vi "test_RPLiDAR_unit-cmd-tester.vi"() -> ()   [LabVIEW 2019]
uses:
  <vilib>/Instr/_visa.llb/VISA Configure Serial Port (Instr).vi
panel:
  out "Waveform Chart":u32(graph)
  out "error out":errorcluster
  in  "clear":bool
  in  "unsigned byte array 9":u8[](array[numeric])=[165, 130, 5, 0, 0, 0, 0, 0, 34] format="%02x"
  in  "unsigned byte array 10":u8[](array[numeric])=[165, 37, 165, 240, 2, 0, 0, 87, 165, 37, 0, 0, 0, 0, 0, 0, 0, 0, 0, 0, 0, 0, 0, 0, 0, 0, 0, 0, 0, 0, 0, 0, 0, 0, 0, 0, 0, 121] format="%02x"
  in  "write 10":bool
  in  "write 9":bool
  in  "84 get lidar conf":u8[](array[numeric])=[165, 132, 36, 117, 0, 0, 0, 1, 0, 0, 0, 0, 0, 0, 0, 0, 0, 0, 0, 0, 0, 0, 0, 0, 0, 0, 0, 0, 0, 0, 0, 0, 0, 0, 0, 0, 0, 0, 113] format="%02x"
  in  "write 8":bool
  in  "25 stop / 50 info":u8[](array[numeric])=[165, 37, 165, 80] format="%02x"
  in  "write 7":bool
  in  "84 get lidar conf":u8[](array[numeric])=[165, 132, 36, 124, 0, 0, 0, 0, 0, 0, 0, 0, 0, 0, 0, 0, 0, 0, 0, 0, 0, 0, 0, 0, 0, 0, 0, 0, 0, 0, 0, 0, 0, 0, 0, 0, 0, 0, 121] format="%02x"
  in  "write 6":bool
  in  "20 get info":u8[](array[numeric])=[165, 80] format="%02x"
  in  "write 5":bool
  in  "motor start":u8[](array[numeric])=[165, 240, 2, 148, 2, 193, 165, 80] format="%02x"
  in  "write 4":bool
  in  "write 3":bool
  in  "get health":u8[](array[numeric])=[165, 82] format="%02x"
  in  "motor stop":u8[](array[numeric])=[165, 240, 2, 0, 0, 87, 165, 80] format="%02x"
  in  "write 2":bool
  in  "dt":u32=10
  in  "write":bool
  in  "unsigned byte array":u8[](array[numeric])=[165, 255, 4, 0, 0, 0, 0, 94] format="%02x"
  out "concatenated string":string
  out "read buffer":string
  in  "stop":bool
  in  "baud rate":u32=115200
  in  "port":refnum<visa-resource-name>="COM6"
  # "A5 20\nA5 52"
  # "RPLidar command tester"
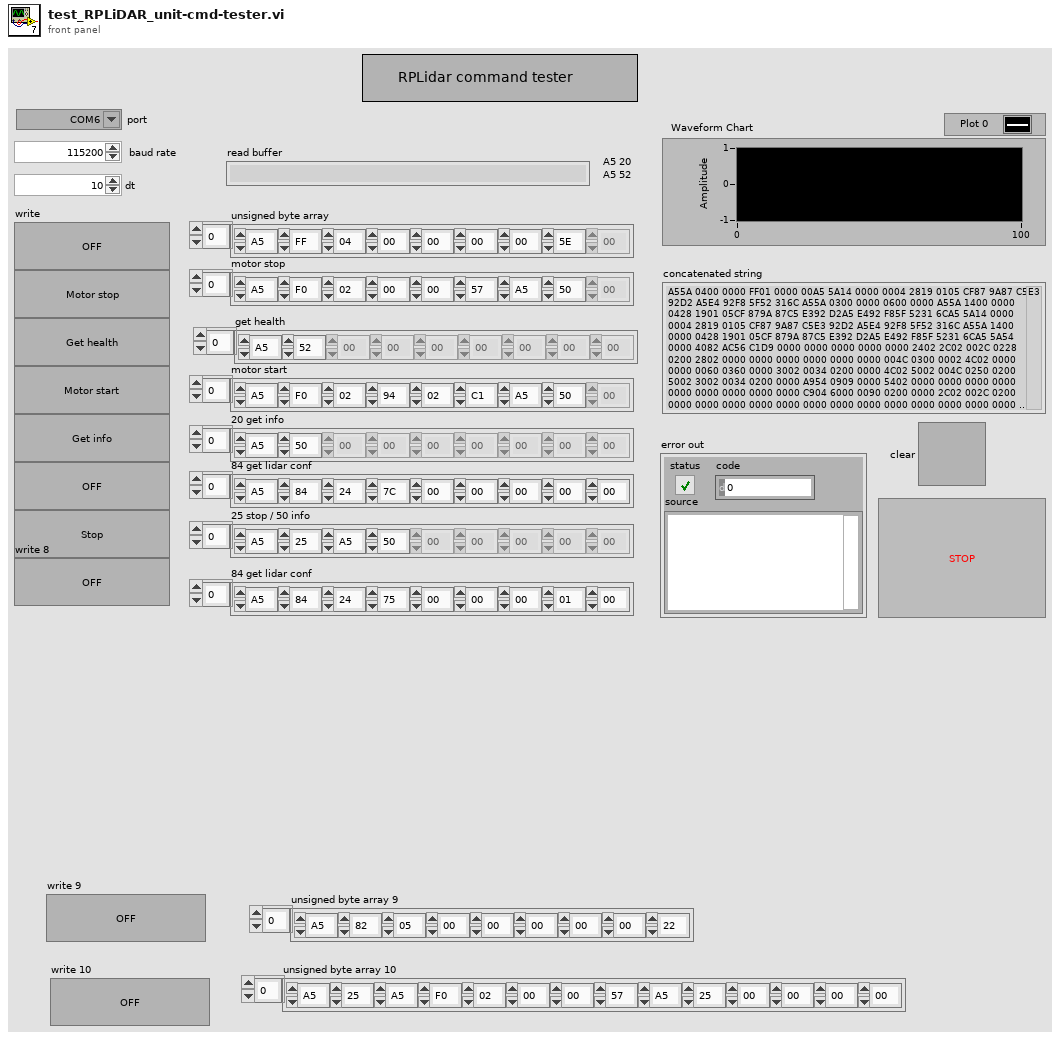
[diagram p1: front panel]
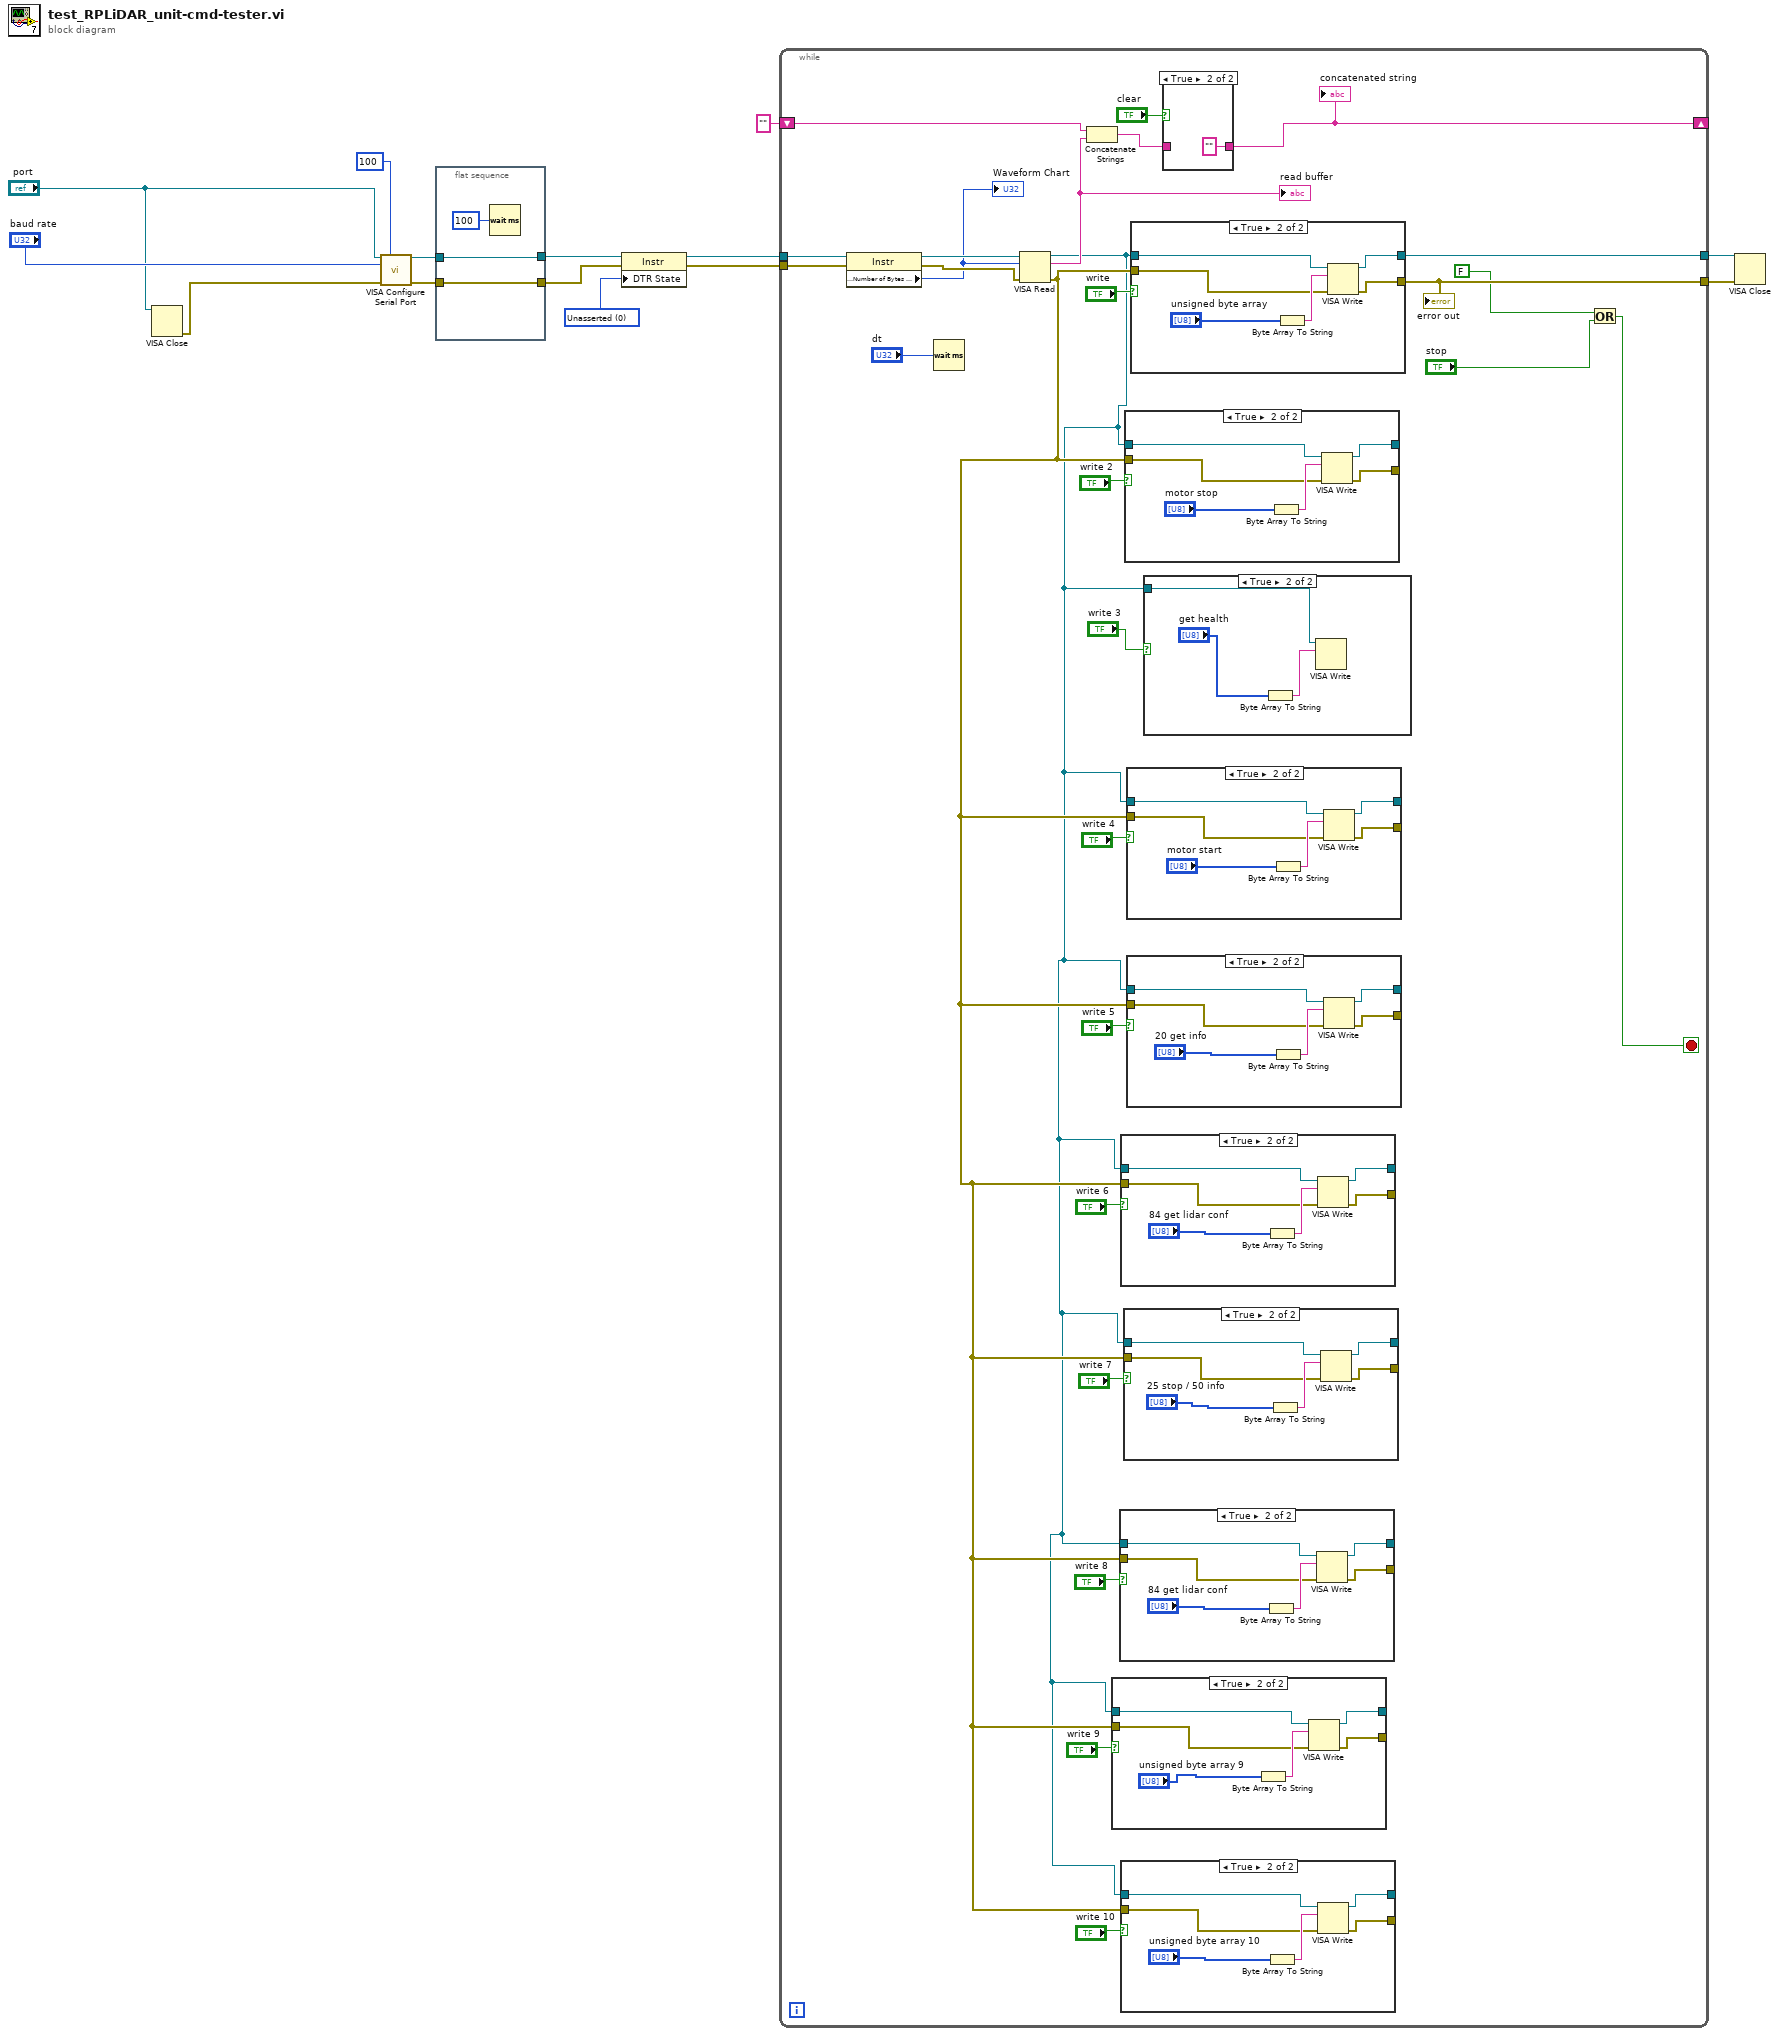
[diagram p0: block diagram]
diagram:
  w9 = i16 0 items=["Unknown"=-1, "Unasserted"=0, "Asserted"=1] ("Serial Settings:Modem Line Settings:Line DTR State")
  n1 = VISA Close(VISA resource name="port") -> (error out=w1:errorcluster)  [unwired: 1 in]
  n2 = call-poly "VISA Configure Serial Port"("VISA resource name"="port", "timeout (10sec)"=u32 100, "baud rate (9600)"="baud rate", "error in (no error)"=w1) -> ("VISA resource name out"=w13:refnum<visa-resource-name>, "error out"=w12:errorcluster)  [unwired: 10 in]
  n3 = flat-sequence {
    tunnel: [w16] -> w11
    tunnel: w13 -> [w16]
    tunnel: [w15] -> w10
    tunnel: w12 -> [w15]
    frame #0 {
      n4 = Wait (ms)(milliseconds to wait=u32 100) -> ()  [unwired: 1 out]
    }
  }
  n5 = property class="Instr"(reference=w11, error in=w10, "DTR State"=w9) -> (reference out=w7:refnum<visa-resource-name>, error out=w6:errorcluster)
  n6 = while {
    tunnel: w7 -> [w45]
    tunnel: w6 -> [w41]
    tunnel: [w39] -> w5
    shift-right: [w20] -> _
    shift-left: "" -> [w42]
    tunnel: [w37] -> w3
    stop <- w35 stop-if-true
    n7 = property class="Instr"(reference=w45, error in=w41) -> (reference out=w44:refnum<visa-resource-name>, error out=w40:errorcluster, "Serial Settings:Number of Bytes at Serial Port"=w18:u32)
    "Waveform Chart" <- w18
    n8 = Wait (ms)(milliseconds to wait="dt") -> ()  [unwired: 1 out]
    n9 = VISA Read(VISA resource name=w44, byte count=w18, error in (no error)=w40) -> (VISA resource name out=w23:refnum<visa-resource-name>, read buffer=w43:string, error out=w25:errorcluster)  [unwired: 1 out]
    "read buffer" <- w43
    n10 = Concatenate Strings(w42, w43) -> (w21:string)
    n11 = case shown="True" "write 9" {
      tunnel: w23 -> [w60 w66]
      tunnel: [w60 w65] -> _
      tunnel: [w59 w63] -> _
      tunnel: w25 -> [w59 w62]
      frame False {
      }
      frame True {
        n12 = Byte Array To String(unsigned byte array="unsigned byte array 9") -> (string=w64:string)
        n13 = VISA Write(VISA resource name=w66, write buffer=w64, error in (no error)=w62) -> (VISA resource name out=w65:refnum<visa-resource-name>, error out=w63:errorcluster)  [unwired: 1 out]
      }
    }
    n14 = case shown="True" "write 8" {
      tunnel: w23 -> [w68 w74]
      tunnel: [w68 w73] -> _
      tunnel: [w67 w71] -> _
      tunnel: w25 -> [w67 w70]
      frame False {
      }
      frame True {
        n15 = Byte Array To String(unsigned byte array="84 get lidar conf") -> (string=w72:string)
        n16 = VISA Write(VISA resource name=w74, write buffer=w72, error in (no error)=w70) -> (VISA resource name out=w73:refnum<visa-resource-name>, error out=w71:errorcluster)  [unwired: 1 out]
      }
    }
    n17 = case shown="True" "write 6" {
      tunnel: w23 -> [w84 w90]
      tunnel: [w84 w89] -> _
      tunnel: [w83 w87] -> _
      tunnel: w25 -> [w83 w86]
      frame False {
      }
      frame True {
        n18 = Byte Array To String(unsigned byte array="84 get lidar conf") -> (string=w88:string)
        n19 = VISA Write(VISA resource name=w90, write buffer=w88, error in (no error)=w86) -> (VISA resource name out=w89:refnum<visa-resource-name>, error out=w87:errorcluster)  [unwired: 1 out]
      }
    }
    n20 = case shown="True" "write 10" {
      tunnel: w23 -> [w52 w58]
      tunnel: [w52 w57] -> _
      tunnel: [w51 w55] -> _
      tunnel: w25 -> [w51 w54]
      frame False {
      }
      frame True {
        n21 = Byte Array To String(unsigned byte array="unsigned byte array 10") -> (string=w56:string)
        n22 = VISA Write(VISA resource name=w58, write buffer=w56, error in (no error)=w54) -> (VISA resource name out=w57:refnum<visa-resource-name>, error out=w55:errorcluster)  [unwired: 1 out]
      }
    }
    n23 = case shown="True" "write 7" {
      tunnel: w23 -> [w76 w82]
      tunnel: [w76 w81] -> _
      tunnel: [w75 w79] -> _
      tunnel: w25 -> [w75 w78]
      frame False {
      }
      frame True {
        n24 = Byte Array To String(unsigned byte array="25 stop / 50 info") -> (string=w80:string)
        n25 = VISA Write(VISA resource name=w82, write buffer=w80, error in (no error)=w78) -> (VISA resource name out=w81:refnum<visa-resource-name>, error out=w79:errorcluster)  [unwired: 1 out]
      }
    }
    n26 = case shown="True" "write 2" {
      tunnel: w23 -> [w108 w114]
      tunnel: [w108 w113] -> _
      tunnel: [w107 w110] -> _
      tunnel: w25 -> [w107 w109]
      frame False {
      }
      frame True {
        n27 = Byte Array To String(unsigned byte array="motor stop") -> (string=w112:string)
        n28 = VISA Write(VISA resource name=w114, write buffer=w112, error in (no error)=w109) -> (VISA resource name out=w113:refnum<visa-resource-name>, error out=w110:errorcluster)  [unwired: 1 out]
      }
    }
    n29 = case shown="True" "write 4" {
      tunnel: w23 -> [w100 w106]
      tunnel: [w100 w105] -> _
      tunnel: [w99 w102] -> _
      tunnel: w25 -> [w99 w101]
      frame False {
      }
      frame True {
        n30 = Byte Array To String(unsigned byte array="motor start") -> (string=w104:string)
        n31 = VISA Write(VISA resource name=w106, write buffer=w104, error in (no error)=w101) -> (VISA resource name out=w105:refnum<visa-resource-name>, error out=w102:errorcluster)  [unwired: 1 out]
      }
    }
    n32 = case shown="True" "write 5" {
      tunnel: w23 -> [w92 w98]
      tunnel: [w92 w97] -> _
      tunnel: [w91 w95] -> _
      tunnel: w25 -> [w91 w94]
      frame False {
      }
      frame True {
        n33 = Byte Array To String(unsigned byte array="20 get info") -> (string=w96:string)
        n34 = VISA Write(VISA resource name=w98, write buffer=w96, error in (no error)=w94) -> (VISA resource name out=w97:refnum<visa-resource-name>, error out=w95:errorcluster)  [unwired: 1 out]
      }
    }
    n35 = case shown="True" "write" {
      tunnel: w23 -> [w116 w122]
      tunnel: [w116 w121] -> w39
      tunnel: [w115 w118] -> w37
      tunnel: w25 -> [w115 w117]
      frame False {
      }
      frame True {
        n36 = Byte Array To String(unsigned byte array="unsigned byte array") -> (string=w120:string)
        n37 = VISA Write(VISA resource name=w122, write buffer=w120, error in (no error)=w117) -> (VISA resource name out=w121:refnum<visa-resource-name>, error out=w118:errorcluster)  [unwired: 1 out]
      }
    }
    "error out" <- w37
    n38 = case shown="True" "write 3" {
      tunnel: w23 -> [_ w48]
      frame False {
      }
      frame True {
        n39 = Byte Array To String(unsigned byte array="get health") -> (string=w50:string)
        n40 = VISA Write(VISA resource name=w48, write buffer=w50) -> ()  [unwired: 1 in, 3 out]
      }
    }
    n41 = case shown="True" "clear" {
      tunnel: w21 -> [w46 _]
      tunnel: [w46 ""] -> w20
      frame False {
      }
      frame True {
      }
    }
    "concatenated string" <- w20
    n42 = Or(x=FALSE, y="stop") -> (x .or. y?=w35:bool)
  }
  n43 = VISA Close(VISA resource name=w5, error in (no error)=w3) -> ()  [unwired: 1 out]
